vi "GetArrCtrlFromClusterCtrl.vi"(11 "cluster in":refnum<vi>) -> (2 "arr ctrl":refnum<vi>[](array[refnum]), 3 "cluster out":refnum<vi>)   [LabVIEW 2018, in "Library-Ctrl.lvlib"]
uses:
  Library-Ctrl.lvlib
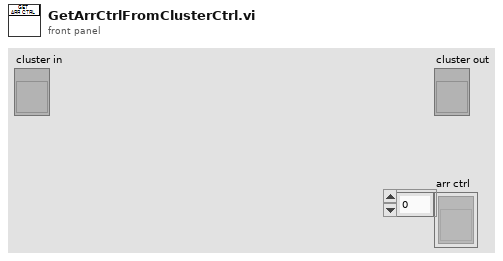
[diagram p1: front panel]
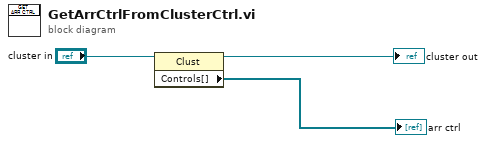
[diagram p0: block diagram]
diagram:
  n1 = property class="Clust"(reference="cluster in") -> (reference out=→"cluster out":refnum<vi>, "Controls[]"=→"arr ctrl":refnum<vi>[])  [unwired: 1 in, 1 out]
